vi "Find Monkey Yelling Number.vi"(0 "Monkey":string, 1 "Monkeys":T1) -> (2 "Monkey Yelling Number":u64)   [LabVIEW 2020, in "AoC 2022.lvlib"]
uses:
  AoC 2022.lvlib
  Day 11 - Monkey in the Middle/private/Monkeys.ctl
  Day 11 - Monkey in the Middle/private/Monkey.ctl
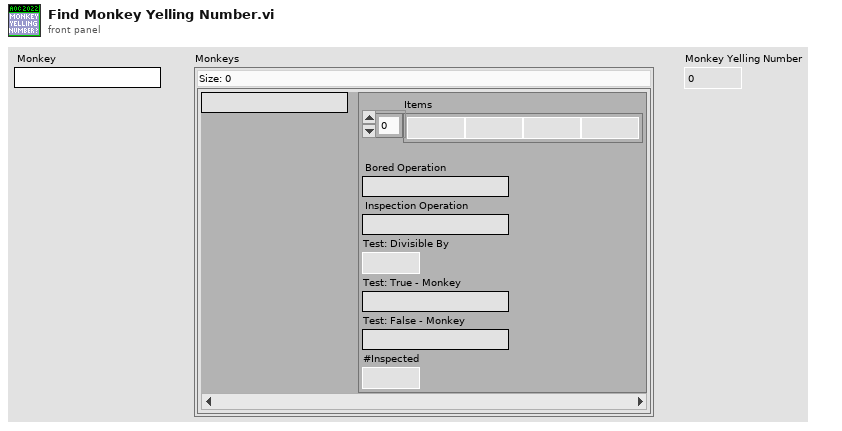
[diagram p1: front panel]
types:
  T1 = typedef "AoC 2022.lvlib/Monkeys.ctl" = map{string, T2}
  T2 = typedef "AoC 2022.lvlib/Monkey.ctl" = cluster{"Items":u64[], "Bored Operation":string, "Inspection Operation":string, "Test: Divisible By":u64, "Test: True - Monkey":string, "Test: False - Monkey":string, "#Inspected":i32}
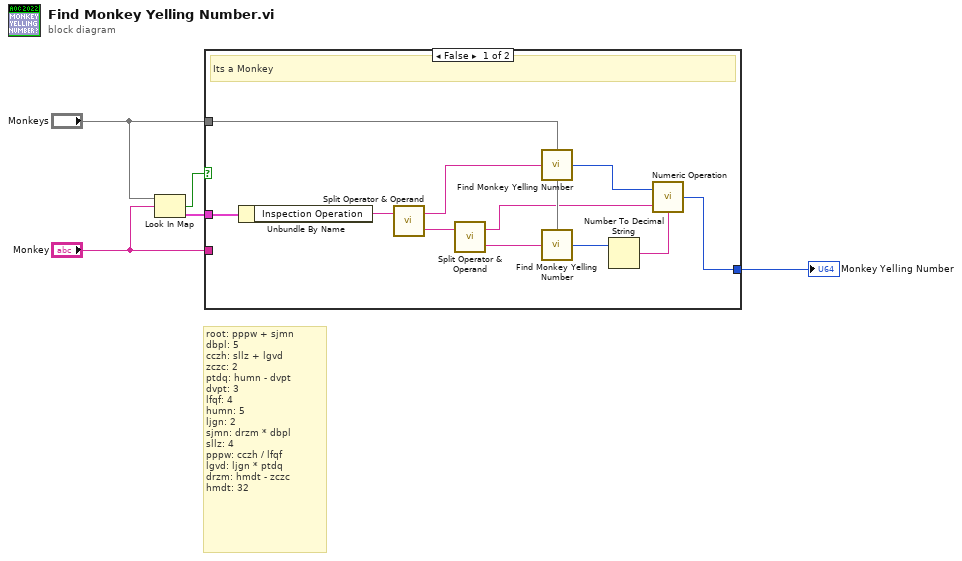
[diagram p0: block diagram]
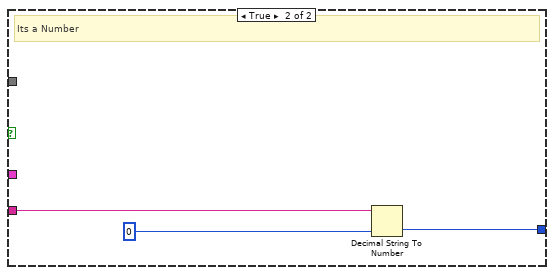
[diagram p2: hidden frame]
diagram:
  # "root: pppw + sjmn\ndbpl: 5\ncczh: sllz + lgvd\nzczc: 2\nptdq: humn - dvpt\ndvpt: 3\nlfqf: 4\nhumn: 5\nljgn: 2\nsjmn: drzm * dbpl\nsllz: 4\npppw: cczh / lfqf\nlgvd: ljgn * ptdq\ndrzm: hmdt - zczc\nhmdt: 32"
  n1 = Look In Map(map="Monkeys", key="Monkey") -> (key not found?=w4:bool, value=w5:T2)  [unwired: 1 in]
  n2 = case shown="False" w4 {
    tunnel: w5 -> [w15 _]
    tunnel: "Monkey" -> [_ w19]
    tunnel: [w6 w18] -> w2
    tunnel: "Monkeys" -> [w11 _]
    frame False {
      # "Its a Monkey"
      n3 = Unbundle By Name(w15) -> ("Inspection Operation"=w16:string)
      n4 = call "Split Operator & Operand.vi"("Operation"=w16) -> ("Operand"=w13:string, "Operator"=w14:string)  [unwired: 1 in]
      n5 = call "Split Operator & Operand.vi"("Operation"=w13) -> ("Operand"=w12:string, "Operator"=w9:string)  [unwired: 1 in]
      n6 = call "Find Monkey Yelling Number.vi"("Monkey"=w14, "Monkeys"=w11) -> ("Monkey Yelling Number"=w10:u64)
      n7 = call "Find Monkey Yelling Number.vi"("Monkey"=w12, "Monkeys"=w11) -> ("Monkey Yelling Number"=w8:u64)
      n8 = Number To Decimal String(number=w8) -> (decimal integer string=w7:string)  [unwired: 1 in]
      n9 = call "Numeric Operation.vi"("Operand 2"=w7, "Operator"=w9, "Operand 1"=w10) -> ("Result"=w6:u64)
    }
    frame True {
      # "Its a Number"
      n10 = Decimal String To Number(string=w19, default (0L)=u64 0) -> (number=w18:u64)  [unwired: 1 in, 1 out]
    }
  }
  "Monkey Yelling Number" <- w2
